vi "Initialization VI.vi"(8 "error in (no error)":errorcluster, 10 "Custom XML":string, 11 "Device Item Ref in":T1 format="%.0x") -> (0 "error out":errorcluster, 3 "Device Item Ref out":T1 format="%.0x")   [LabVIEW 2015, in "J1939 Addon System Explorer.lvlib"]
uses:
  J1939 Addon System Explorer.lvlib
  <vilib>/NI Veristand/Custom Device API/Custom Device Item Ref.ctl
  Shared/SubVIs/Constants.vi
  <vilib>/NI Veristand/Custom Device API/Set Item Property (Variant).vi
  Shared/J1939 Addon Shared.lvlib
  <vilib>/NI Veristand/Custom Device API/Custom Device API.lvlib
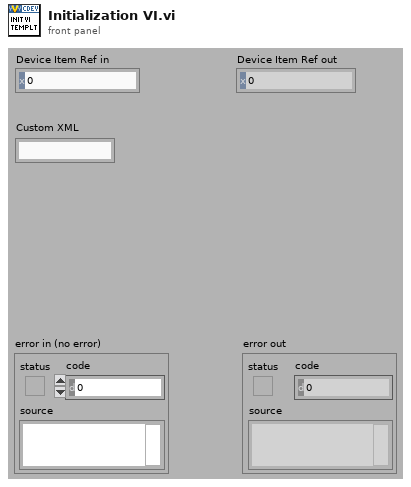
[diagram p1: front panel]
types:
  T1 = typedef "Custom Device API.lvlib/Custom Device Item Ref.ctl" = u64
  T2 = typedef "J1939 Addon Shared.lvlib/Monitor Settings.ctl" = cluster{"J1939 Network Address":u8, "Name":u64}
  T3 = typedef "J1939 Addon Shared.lvlib/XNET Settings.ctl" = cluster{"XNET Database":refnum<k21>, "XNET Cluster":refnum<k21>, "CAN Port":string, "Baud rate [Bd]":u32, "Termination":u32, "Incoming Rate":u32, "Outcoming Rate":u32, "Write Decimation":u32}
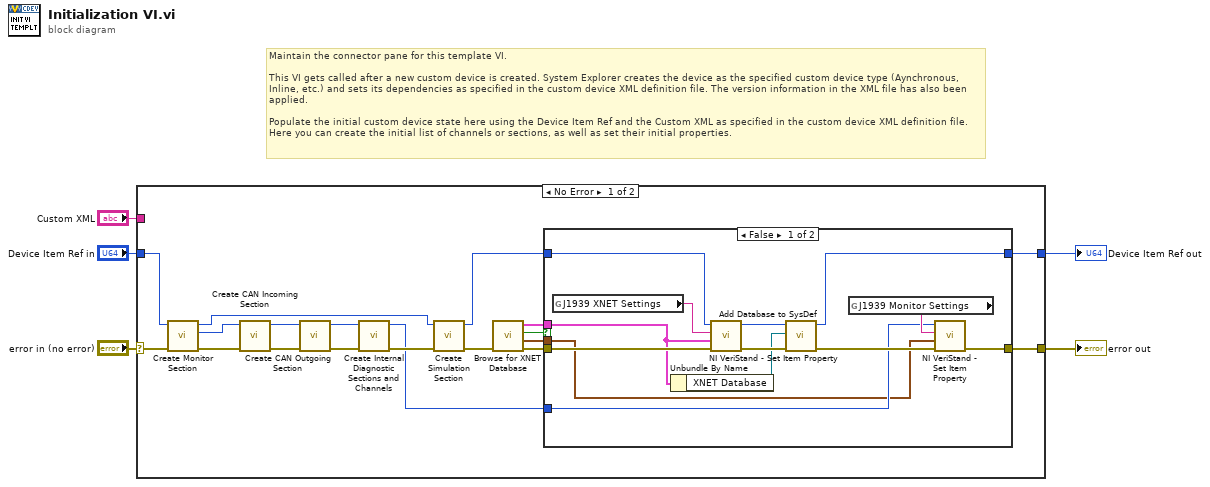
[diagram p0: block diagram]
diagram:
  # "Maintain the connector pane for this template VI.\n\nThis VI gets called after a new custom device is created. System Explorer creates the device as the specified custom device type (Aynchronous, Inline, etc.) and sets its dependencies as specified in the custom device XML definition file. The version information in the XML file has also been applied.\n\nPopulate the initial custom device state here using the Device Item Ref and the Custom XML as specified in the custom device XML definition file. Here you can create the initial list of channels or sections, as well as set their initial properties."
  n1 = case shown="No Error" "error in (no error)" {
    selector: "error in (no error)" -> [w13 w41]
    tunnel: [w22 w41] -> w5
    tunnel: [w18 w40] -> w3
    tunnel: "Device Item Ref in" -> [w11 w40]
    tunnel: "Custom XML" -> [_ _]
    frame No Error {
      n2 = call "Create Monitor Section.vi"("error in (no error)"=w13, "Device Item Ref in"=w11) -> ("error out"=w12:errorcluster, "Section Ptr"=w6:T1, "Parent Ref out"=w7:T1)  [unwired: 7 in]
      n3 = call "Create CAN Incoming Section.vi"("error in (no error)"=w12, "Device Item Ref in"=w6) -> ("error out"=w24:errorcluster, "Device Item Ref Out"=w23:T1)  [unwired: 8 in]
      n4 = call "Create CAN Outgoing Section.vi"("error in (no error)"=w24, "Parent Ref in"=w23) -> ("error out"=w16:errorcluster, "Parent Ref out"=w17:T1)  [unwired: 8 in]
      n5 = call "Create Internal Diagnostic Sections and Channels.vi"("error in (no error)"=w16, "Device Item Ref in"=w17) -> ("error out"=w15:errorcluster, "Device Item Ref Out"=w8:T1)  [unwired: 8 in]
      n6 = call "Create Simulation Section.vi"("error in (no error)"=w15, "Parent Ref in"=w7) -> ("error out"=w14:errorcluster, "Parent Ref out"=w10:T1)  [unwired: 7 in, 1 out]
      n7 = call "Browse for XNET Database.vi"("error in (no error)"=w14) -> ("error out"=w21:errorcluster, "J1939 Monitor Settings"=w9:T2, "Cancel Out"=w20:bool, "J1939 XNET Settings"=w19:T3)  [unwired: 7 in]
      n8 = case shown="False" w20 {
        tunnel: [w27 w39] -> w22
        tunnel: w21 -> [w37 w39]
        tunnel: w19 -> [w31 _]
        tunnel: w10 -> [w36 w38]
        tunnel: [w32 w38] -> w18
        tunnel: w9 -> [w25 _]
        tunnel: w8 -> [w26 _]
        frame False {
          n9 = global read "Constants.vi" "J1939 XNET Settings"() -> (w35:string)
          n10 = Unbundle By Name(w31) -> ("XNET Database"=w30:refnum<k21>)
          n11 = call-poly <vilib>:"NI VeriStand - Set Item Property.vi"("error in (no error)"=w37, "Value"=w31, "Property Name"=w35, "Item Ref in"=w36) -> ("error out"=w34:errorcluster, "Item Ref out"=w33:T1)  [unwired: 5 in, 1 out]
          n12 = call "Add Database to SysDef.vi"("error in"=w34, "DB Alias"=w30, "Item Ref in"=w33) -> ("error out"=w28:errorcluster, "Item Ref out"=w32:T1)  [unwired: 7 in]
          n13 = global read "Constants.vi" "J1939 Monitor Settings"() -> (w29:string)
          n14 = call-poly <vilib>:"NI VeriStand - Set Item Property.vi"("error in (no error)"=w28, "Value"=w25, "Property Name"=w29, "Item Ref in"=w26) -> ("error out"=w27:errorcluster)  [unwired: 5 in, 2 out]
        }
        frame True {
        }
      }
    }
    frame Error {
    }
  }
  "error out" <- w5
  "Device Item Ref out" <- w3
